vi "Substation.vi"() -> ()   [LabVIEW 2025]
uses:
  <vilib>/numeric/Random Number (Range) U64.vi
  <vilib>/numeric/sub_Random U32.vi
panel:
  out "Ring 2":u16(ring)
  out "Ring":u16(ring)
  in  "Refresh Button":bool
  out "STEP UP":u64(graph)
  out "STEP DOWN":u64(graph)
  out "TURN OFF":bool
  out "Meter":dbl(knob) scale=0.0..10000.0
  out "WARNING 1":bool
  out "LOW TEMP":bool
  out "HIGH TEMP":bool
  out "?":dbl(slide) scale=0.0..5000.0
  out "ITERATION":dbl
  out "I/P VOLT":dbl
  out "STEP UP":bool
  out "STEP DOWN":bool
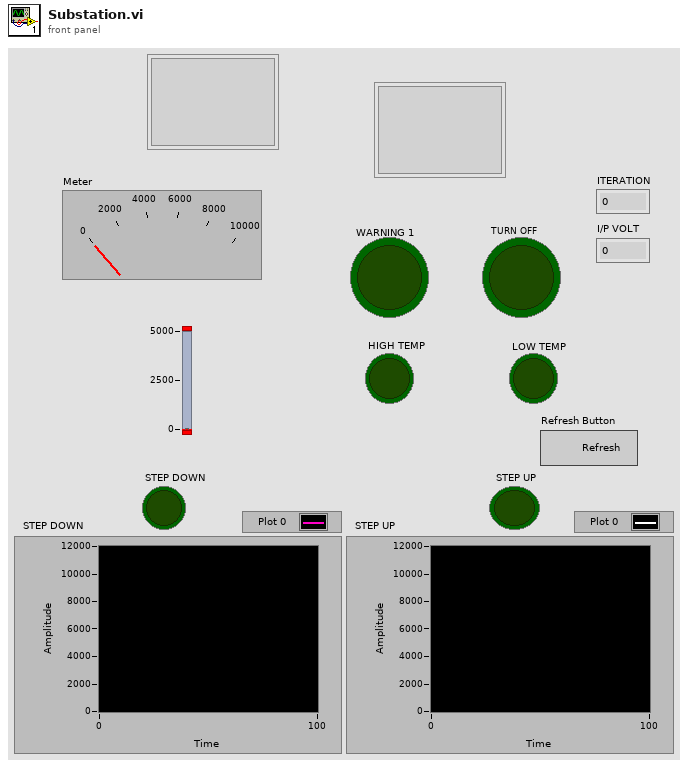
[diagram p1: front panel]
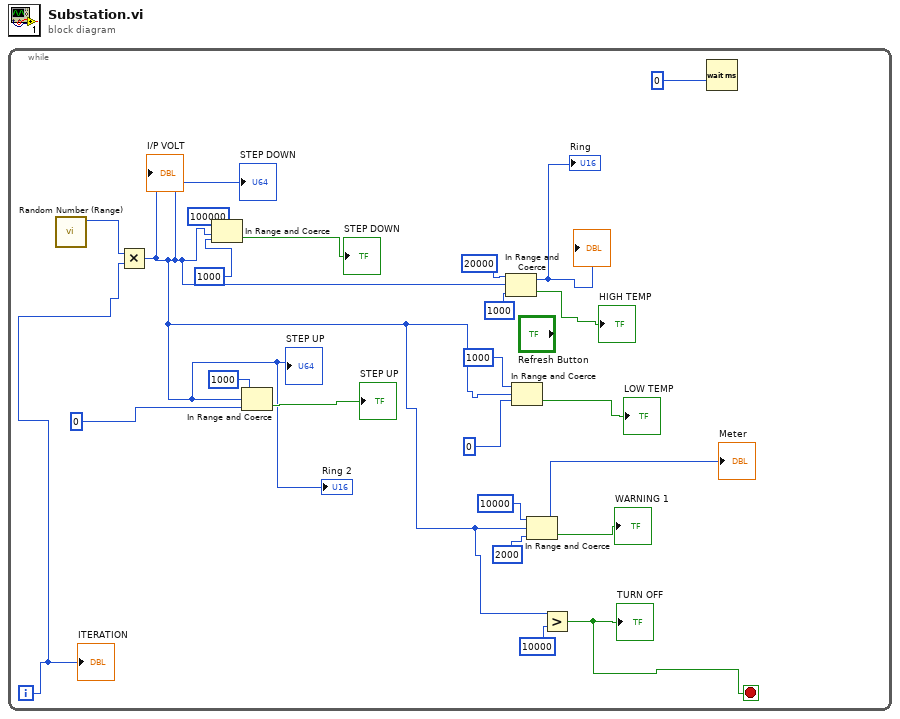
[diagram p0: block diagram]
diagram:
  n1 = while {
    i -> [w4]
    stop <- w7 stop-if-true
    n2 = call-poly <vilib>:"Random Number (Range).vi"() -> ("number"=w3:u64)  [unwired: 11 in]
    n3 = Multiply(x=w3, y=w4) -> (x*y=w1:u64)
    "I/P VOLT" <- w1
    "STEP DOWN" <- w1
    "STEP UP" <- w1
    "Ring 2" <- w1
    n4 = In Range and Coerce(upper limit=100000, x=w1, lower limit=1000) -> (In Range?=→"STEP DOWN":bool)  [unwired: 1 out]
    n5 = In Range and Coerce(upper limit=1000, x=w1, lower limit=0) -> (In Range?=→"STEP UP":bool)  [unwired: 1 out]
    n6 = In Range and Coerce(upper limit=20000, x=w1, lower limit=1000) -> (coerced(x)=→"?" →"Ring":u64, In Range?=→"HIGH TEMP":bool)
    n7 = In Range and Coerce(upper limit=1000, x=w1, lower limit=0) -> (In Range?=→"LOW TEMP":bool)  [unwired: 1 out]
    n8 = In Range and Coerce(upper limit=10000, x=w1, lower limit=2000) -> (coerced(x)=→"Meter":u64, In Range?=→"WARNING 1":bool)
    n9 = Greater?(x=w1, y=10000) -> (0:w7:bool)
    "TURN OFF" <- w7
    n10 = Wait (ms)(milliseconds to wait=0) -> ()  [unwired: 1 out]
    "ITERATION" <- w4
  }
